vi "Logging_LogValues.vi"(8 "error in":errorcluster, 10 "Column Values":dbl[](array[numeric]), 11 "Byte Stream File in":refnum<file>) -> (0 "error out":errorcluster, 3 "Byte Stream File out":refnum<file>)   [LabVIEW 2014]
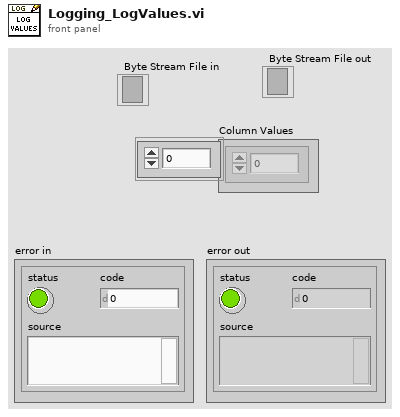
[diagram p1: front panel]
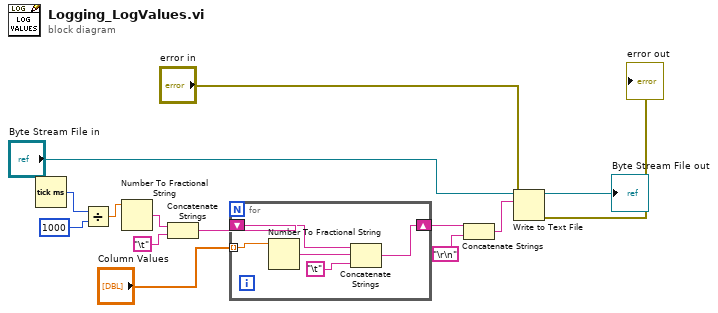
[diagram p0: block diagram]
diagram:
  n1 = Tick Count (ms)() -> (millisecond timer value=w5:u32)
  n2 = Divide(x=w5, y=1000) -> (x/y=w7:dbl)
  n3 = Number To Fractional String(number=w7) -> (F-format string=w4:string)  [unwired: 3 in]
  n4 = Concatenate Strings(w4, "\t") -> (w10:string)
  n5 = for {
    tunnel: "Column Values" -> [w19] mode=indexing
    shift-right: [w15] -> w11
    shift-left: w10 -> [w16]
    n6 = Number To Fractional String(number=w19) -> (F-format string=w18:string)  [unwired: 3 in]
    n7 = Concatenate Strings(w16, w18, "\t") -> (w15:string)
  }
  n8 = Concatenate Strings(w11, "\r\n") -> (w13:string)
  n9 = Write to Text File(file (use dialog)="Byte Stream File in", text=w13, error in="error in") -> (refnum out=→"Byte Stream File out":refnum<file>, error out=→"error out":errorcluster)  [unwired: 1 in, 1 out]
